vi "Get Domain.vi"(8 "error in (no error)":errorcluster, 11 "Domain_Steady_2D_Polygon in":refnum<class "NI_Domain_Steady_2D_Polygon.lvclass">) -> (0 "error out":errorcluster, 2 "domain":variant, 3 "Domain_Steady_2D_Polygon out":refnum<class "NI_Domain_Steady_2D_Polygon.lvclass">)   [LabVIEW 2020, in "NI_PDE.lvlib" / "NI_Domain_Steady_2D_Polygon.lvclass"]
uses:
  <vilib>/gmath/pde.llb/DomainClass/Domain_Steady_2D_Polygon/NI_Domain_Steady_2D_Polygon.lvclass
  <vilib>/gmath/pde.llb/DomainClass/Domain_Steady_2D_Polygon/Domain Data.ctl
  <vilib>/gmath/pde.llb/DomainClass/Domain_Steady_2D_Polygon/NI_Domain_Steady_2D_Polygon.lvclass/NI_Domain_Steady_2D_Polygon.ctl
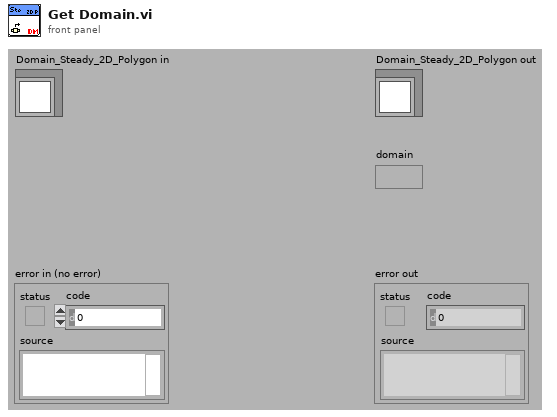
[diagram p1: front panel]
types:
  T1 = typedef "NI_PDE.lvlib/NI_Domain_Steady_2D_Polygon.lvclass/Domain Data.ctl" = cluster{"X":dbl[], "Y":dbl[], "Xi":dbl[], "Yi":dbl[], "grid factor":dbl, "Triangulation":i32[][]}
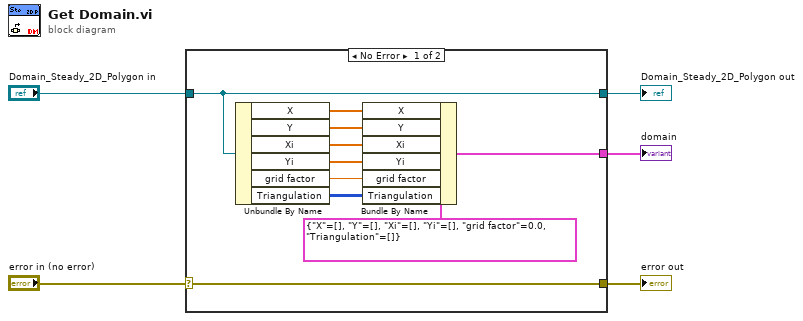
[diagram p0: block diagram]
diagram:
  n1 = case shown="No Error" "error in (no error)" {
    selector: "error in (no error)" -> [w6 w17]
    tunnel: "Domain_Steady_2D_Polygon in" -> [w13 w16]
    tunnel: [w13 w16] -> w5
    tunnel: [w6 w17] -> w4
    tunnel: [w14 _] -> w1
    frame No Error {
      n2 = Unbundle By Name(w13) -> ("X"=w12:dbl[], "Y"=w11:dbl[], "Xi"=w10:dbl[], "Yi"=w9:dbl[], "grid factor"=w8:dbl, "Triangulation"=w7:i32[][])
      n3 = Bundle By Name(cluster=T1 {"X"=[], "Y"=[], "Xi"=[], "Yi"=[], "grid factor"=0.0, "Triangulation"=[]} ("domain data"), "X"=w12, "Y"=w11, "Xi"=w10, "Yi"=w9, "grid factor"=w8, "Triangulation"=w7) -> (w14:T1)
    }
    frame Error {
    }
  }
  "Domain_Steady_2D_Polygon out" <- w5
  "error out" <- w4
  "domain" <- w1
